vi "Test Process Lifecycle States.vi"(8 "error in (no error)":errorcluster, 11 "Process Test In":refnum<class "Process Dev Test.lvclass">) -> (0 "error out":errorcluster, 3 "Process Test Out":refnum<class "Process Dev Test.lvclass">)   [LabVIEW 2020, in "Process Dev Test.lvclass"]
uses:
  Process Dev Test.lvclass
  C:/Program Files (x86)/National Instruments/LabVIEW 2020/vi.lib/Astemes/LUnit/Test Case.lvclass
  source/Framework/Process/Public/Lifecycle/Lifecycle State.ctl
  source/Framework/Process/Process.lvclass/Process.ctl
  <vilib>/Astemes/LUnit/Test Case.lvclass/Test Case.ctl
  <vilib>/Astemes/LUnit/LUnit Assertion Result.lvclass/LUnit Assertion Result.ctl
  <vilib>/Astemes/LUnit/LUnit Test Case Result.lvclass/LUnit Test Case Result.ctl
  <vilib>/Astemes/LUnit/LUnit Method Result.lvclass/LUnit Method Result.ctl
  <vilib>/Utility/error.llb/Clear Errors.vi
  <vilib>/Astemes/LUnit/Palette/Fail.vi
  <vilib>/Astemes/LUnit/Palette/Pass.vi
  <vilib>/Astemes/LUnit/Set Assertion Type.vi
  source/Framework/Process/Private/SubVIs/Wait for finish.vi
  source/Framework/Process/Protected/Messaging/Enqueue Message.vi
  source/Framework/Process/Private/SubVIs/Set Lifecycle State.vi
  <vilib>/Astemes/LUnit/Add test result.vi
  <vilib>/Astemes/LUnit/LUnit Write Passed.vi
  <vilib>/Astemes/LUnit/LUnit Write Message.vi
  <vilib>/Astemes/LUnit/LUnit Write Description.vi
  <vilib>/Astemes/LUnit/LUnit Write Assertion Type.vi
  source/Framework/Process/Private/SubVIs/Handle Debug Data.vi
  <vilib>/Astemes/LUnit/LUnit Record Assertion Result.vi
  source/Framework/Logging/Log Debug.vi
  <vilib>/AdvancedString/1D String Array to Delimited String.vi
  <vilib>/Utility/High Resolution Relative Seconds.vi
  <vilib>/Astemes/LUnit/LUnit Aggregate Assertion Results.vi
  <vilib>/Astemes/LUnit/Assertion Result/LUnit Read Status.vi
  <vilib>/Astemes/LUnit/LUnit Read Message.vi
  <vilib>/Astemes/LUnit/LUnit Read Description.vi
  <vilib>/Astemes/LUnit/Method Result/LUnit Merge Status.vi
  <vilib>/Astemes/LUnit/LUnit Concatenate result strings.vi
  <vilib>/Utility/error.llb/Error Cluster From Error Code.vi
  source/Framework/Process/Public/Read Name.vi
  <vilib>/Astemes/LUnit/LUnit Assertion Result.lvclass
  source/Framework/Process/Process.lvclass
  <vilib>/Astemes/LUnit/Test Case.lvclass
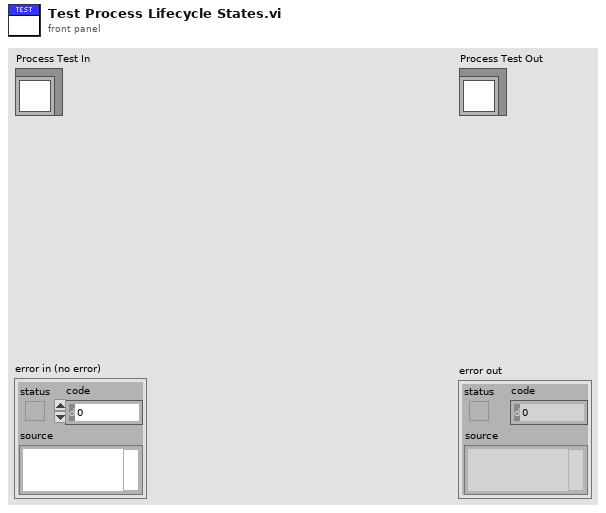
[diagram p1: front panel]
types:
  T1 = typedef "Process.lvclass/Lifecycle State.ctl" = enum16{"Uninitialized", "Initialized", "Started", "Running", "Stopped", "Finished"}
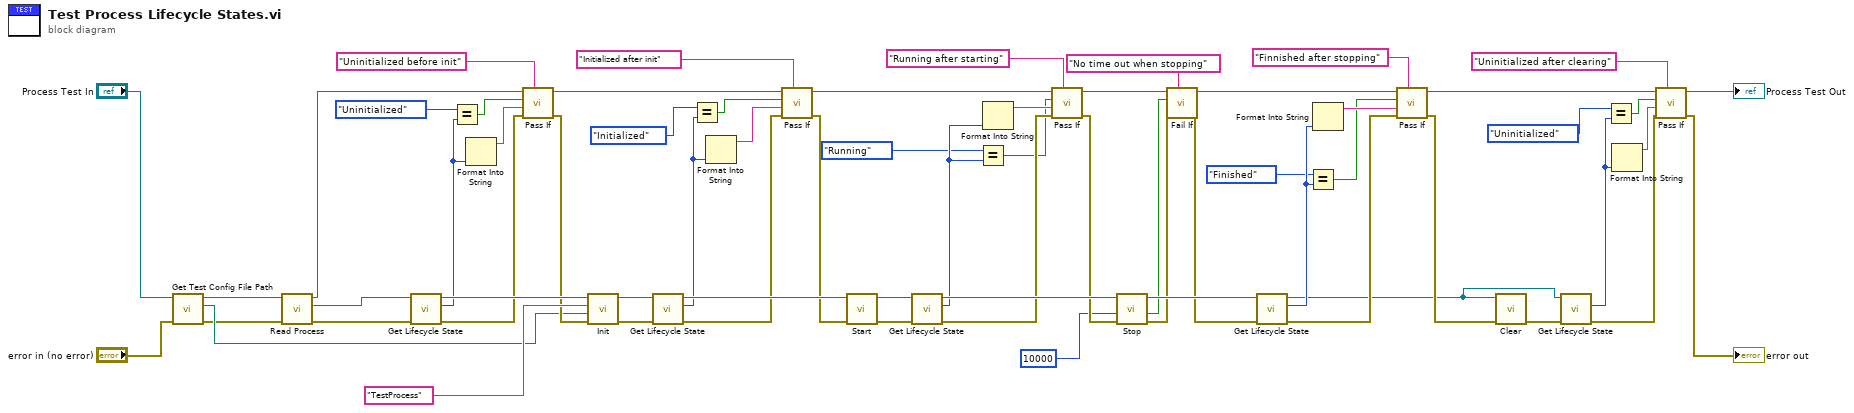
[diagram p0: block diagram]
diagram:
  n1 = call "Get Test Config File Path.vi"("error in (no error)"="error in (no error)", "Process Test In"="Process Test In") -> ("error out"=w11:errorcluster, "Test config path"=w30:path, "Process Test Out"=w13:refnum<class "Process Dev Test.lvclass">)  [unwired: 7 in]
  n2 = call "Read Process.vi"("error in (no error)"=w11, "Process Test in"=w13) -> ("error out"=w10:errorcluster, "Process.lvclass"=w12:refnum<class "Process.lvclass">, "Process Test out"=w8:refnum<class "Process Dev Test.lvclass">)  [unwired: 7 in]
  n3 = call "Get Lifecycle State.vi"("error in (no error)"=w10, "Process In"=w12) -> ("error out"=w51:errorcluster, "Lifecycle State"=w26:T1, "Process Out"=w65:refnum<class "Process.lvclass">)  [unwired: 6 in, 1 out]
  n4 = Equal?(x=Lifecycle_State."Uninitialized" ("Lifecycle State"), y=w26) -> (x = y?=w25:bool)
  n5 = Format Into String(w26) -> (resulting string=w24:string)  [unwired: 3 in, 1 out]
  n6 = call <vilib>:"Pass If.vi"("Description"="Uninitialized before init", "error in (no error)"=w51, "Message"=w24, "Pass?"=w25, "LUnit Test Case In"=w8) -> ("error out"=w50:errorcluster, "LUnit Test Case Out"=w55:refnum<class "Process Dev Test.lvclass">)  [unwired: 5 in]
  n7 = call-dynamic "Init.vi"("error in (no error)"=w50, "Config File Path"=w30, "Name"="TestProcess", "Process In"=w65) -> ("error out"=w63:errorcluster, "Process Out"=w64:refnum<class "Process.lvclass">)  [unwired: 6 in]
  n8 = call "Get Lifecycle State.vi"("error in (no error)"=w63, "Process In"=w64) -> ("error out"=w49:errorcluster, "Lifecycle State"=w29:T1, "Process Out"=w62:refnum<class "Process.lvclass">)  [unwired: 6 in, 1 out]
  n9 = Equal?(x=Lifecycle_State."Initialized" ("Lifecycle State"), y=w29) -> (x = y?=w28:bool)
  n10 = Format Into String(w29) -> (resulting string=w27:string)  [unwired: 3 in, 1 out]
  n11 = call <vilib>:"Pass If.vi"("Description"="Initialized after init", "error in (no error)"=w49, "Message"=w27, "Pass?"=w28, "LUnit Test Case In"=w55) -> ("error out"=w48:errorcluster, "LUnit Test Case Out"=w54:refnum<class "Process Dev Test.lvclass">)  [unwired: 5 in]
  n12 = call "Start.vi"("error in (no error)"=w48, "Process In"=w62) -> ("error out"=w60:errorcluster, "Process Out"=w61:refnum<class "Process.lvclass">)  [unwired: 7 in, 1 out]
  n13 = call "Get Lifecycle State.vi"("error in (no error)"=w60, "Process In"=w61) -> ("error out"=w47:errorcluster, "Lifecycle State"=w37:T1, "Process Out"=w59:refnum<class "Process.lvclass">)  [unwired: 6 in, 1 out]
  n14 = Equal?(x=Lifecycle_State."Running" ("Lifecycle State"), y=w37) -> (x = y?=w19:bool)
  n15 = Format Into String(w37) -> (resulting string=w36:string)  [unwired: 3 in, 1 out]
  n16 = call <vilib>:"Pass If.vi"("Description"="Running after starting", "error in (no error)"=w47, "Message"=w36, "Pass?"=w19, "LUnit Test Case In"=w54) -> ("error out"=w46:errorcluster, "LUnit Test Case Out"=w53:refnum<class "Process Dev Test.lvclass">)  [unwired: 5 in]
  n17 = call "Stop.vi"("error in (no error)"=w46, "timeout in ms (-1)"=10000, "Process In"=w59) -> ("error out"=w15:errorcluster, "timed out?"=w17:bool, "Process Out"=w58:refnum<class "Process.lvclass">)  [unwired: 6 in]
  n18 = call <vilib>:"Fail If.vi"("Description"="No time out when stopping", "error in (no error)"=w15, "Fail?"=w17, "LUnit Test Case In"=w53) -> ("error out"=w14:errorcluster, "LUnit Test Case Out"=w18:refnum<class "Process Dev Test.lvclass">)  [unwired: 6 in]
  n19 = call "Get Lifecycle State.vi"("error in (no error)"=w14, "Process In"=w58) -> ("error out"=w45:errorcluster, "Lifecycle State"=w34:T1, "Process Out"=w1:refnum<class "Process.lvclass">)  [unwired: 6 in, 1 out]
  n20 = Equal?(x=Lifecycle_State."Finished" ("Lifecycle State"), y=w34) -> (x = y?=w20:bool)
  n21 = Format Into String(w34) -> (resulting string=w33:string)  [unwired: 3 in, 1 out]
  n22 = call <vilib>:"Pass If.vi"("Description"="Finnished after stopping", "error in (no error)"=w45, "Message"=w33, "Pass?"=w20, "LUnit Test Case In"=w18) -> ("error out"=w44:errorcluster, "LUnit Test Case Out"=w52:refnum<class "Process Dev Test.lvclass">)  [unwired: 5 in]
  n23 = call-dynamic "Clear.vi"("error in (no error)"=w44, "Process In"=w1) -> ("error out"=w57:errorcluster)  [unwired: 9 in]
  n24 = call "Get Lifecycle State.vi"("error in (no error)"=w57, "Process In"=w1) -> ("error out"=w43:errorcluster, "Lifecycle State"=w22:T1)  [unwired: 6 in, 2 out]
  n25 = Equal?(x=Lifecycle_State."Uninitialized" ("Lifecycle State"), y=w22) -> (x = y?=w23:bool)
  n26 = Format Into String(w22) -> (resulting string=w21:string)  [unwired: 3 in, 1 out]
  n27 = call <vilib>:"Pass If.vi"("Description"="Uninitialized after clearing", "error in (no error)"=w43, "Message"=w21, "Pass?"=w23, "LUnit Test Case In"=w52) -> ("error out"=→"error out":errorcluster, "LUnit Test Case Out"=→"Process Test Out":refnum<class "Process Dev Test.lvclass">)  [unwired: 5 in]
